vi "Drive for Distance.vi"(5 "speed":dbl, 7 "Distance (ft)":dbl, 11 "Command Info In":T1, 12 "Synchronication":enum16{"Start", "Wait"}(ring)=enum."Wait") -> (15 "Command Info Out":T1)   [LabVIEW 2016]
doc: "This VI notifies the subsystem to the new setpoint."
uses:
  <vilib>/Rock Robotics/WPI/Framework/Command Status Info.ctl
  <vilib>/Rock Robotics/WPI/Framework/Completion Status.ctl
  <vilib>/Rock Robotics/WPI/Framework/Completion Notifier.ctl
  Implementation/Drive Setpoints.ctl
  Implementation/Drive Operations.ctl
panel:
  in  "Description":string
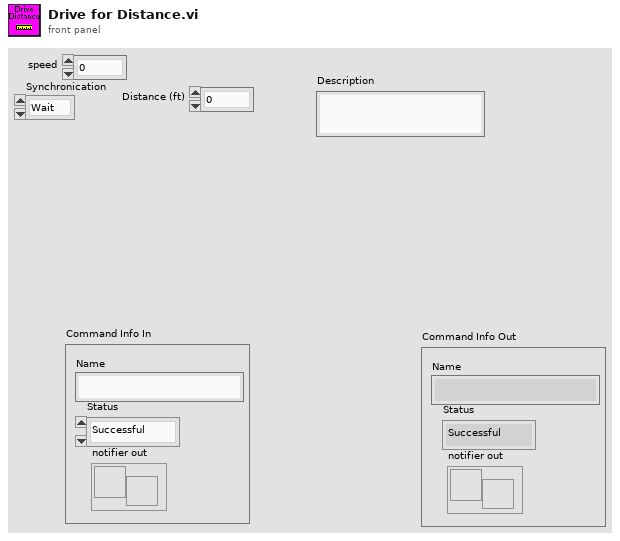
[diagram p1: front panel]
types:
  T1 = typedef "Command Status Info.ctl" = cluster{"Name":string, "Status":T2, "notifier out":T3}
  T2 = typedef "Completion Status.ctl" = enum16{"Successful", "Aborted", "Incomplete"}
  T3 = typedef "Completion Notifier.ctl" = refnum<notifier>
  T4 = typedef "Drive Setpoints.ctl" = cluster{"Operation":T5, "Left Setpoint":dbl, "Right Setpoint":dbl, "Duration":dbl, "Shift state":i8, "Angle":dbl, "Brake":bool}
  T5 = typedef "Drive Operations.ctl" = enum16{"Reserve", "Read Current", "Immediate", "Drive for Time", "Drive for Distance", "Turn to angle", "Vision Turn", "Vision close distance", "Reset Gyro", "Turn until target", "Brake", "DriveStraight"}
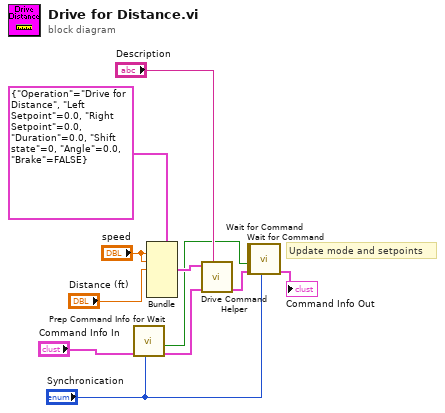
[diagram p0: block diagram]
diagram:
  # "Update mode and setpoints"
  n1 = call <vilib>:"Prep Command Info for Wait.vi"("Synchronication"="Synchronication", "Command Info"="Command Info In") -> ("Command Info"=w4:T1, "Allocated"=w1:bool)  [unwired: 8 in]
  n2 = Bundle(cluster=T4 {"Operation"=enum."Drive for Distance", "Left Setpoint"=0.0, "Right Setpoint"=0.0, "Duration"=0.0, "Shift state"=0, "Angle"=0.0, "Brake"=FALSE} ("SubSystem Data"), "Left Setpoint"="speed", "Right Setpoint"="speed", "Duration"="Distance (ft)") -> (w9:T4)  [unwired: 4 in]
  n3 = call "Drive Command Helper.vi"("Description"="Description", "Command Info In"=w4, "SubSystem Data"=w9) -> ("Command Info Out"=w3:T1)  [unwired: 7 in, 1 out]
  n4 = call <vilib>:"Wait for Command.vi"() -> ()  [unwired: 11 in, 1 out]
  n5 = call <vilib>:"Wait for Command.vi"("Synchronication"="Synchronication", "Command Info in"=w3, "Allocated"=w1) -> ("Command Info out"=→"Command Info Out":T1)  [unwired: 8 in]
